vi "En-queue RT message element.vi"(8 "Data":variant, 9 "Message":string, 11 "RT Queues":T1) -> (3 "RT Queues out":T1)   [LabVIEW 2018]
uses:
  Type Defs/Queues cluster.ctl
  ICL-LabVIEW_General/Message Scheduler/message scheduler.lvclass
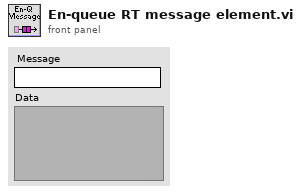
[diagram p1: front panel]
types:
  T1 = typedef "Queues cluster.ctl" = cluster{"RT Message":refnum<queue>, "RT Comms":refnum<queue>, "RT Data":refnum<queue>, "RT FIFO":refnum<queue>, "message scheduler":refnum<class "message scheduler.lvclass">}
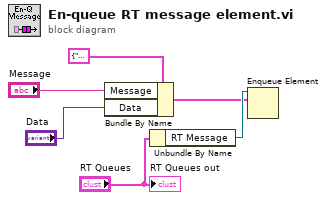
[diagram p0: block diagram]
diagram:
  n1 = Bundle By Name(cluster=cluster{"Message":string, "Data":variant} {"Message"="", "Data"=variant} ("element"), "Message"="Message", "Data"="Data") -> (w3:cluster{"Message":string, "Data":variant})
  n2 = Unbundle By Name("RT Queues") -> ("RT Message"=w5:refnum<queue>)
  n3 = Enqueue Element(queue=w5, element=w3) -> ()  [unwired: 2 in, 3 out]
  "RT Queues out" <- "RT Queues"
